vi "ADC_Abort.vi"(8 "error in (no error)":errorcluster) -> (0 "error out":errorcluster, 3 "function return":i16)   [LabVIEW 2013, in "MeasurmentRoutines.lvlib"]
doc: "Description: This routine aborts a running measurement. Any measured datais lost. It is not required to abort a running measurement before starting a new one, ADC_Start does this already.\nInput: -\nOutput: Return value E_NOT_INITIALIZED | E_NO_ERRORS | E_NO_HARDWARE\n\nFunction prototype: word ADC_Abort( void )\n\n\nshort int ADC_Abort ( void );"
uses:
  MeasurmentRoutines.lvlib
  hs3.dll
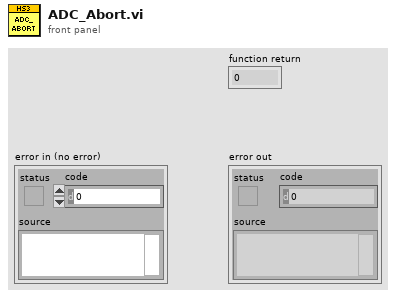
[diagram p1: front panel]
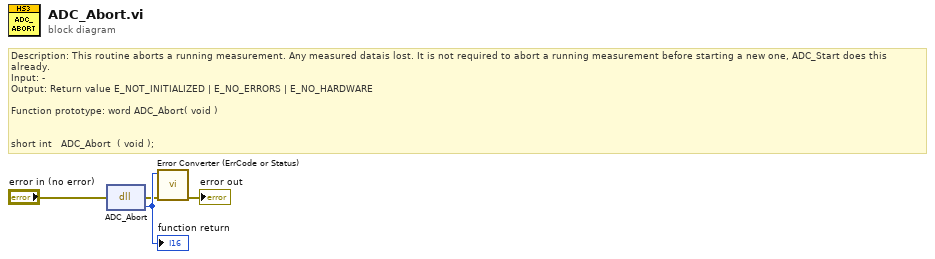
[diagram p0: block diagram]
diagram:
  # "Description: This routine aborts a running measurement. Any measured datais lost. It is not required to abort a running measurement before starting a new one, ADC_Start does this already.\nInput: -\nOutput: Return value E_NOT_INITIALIZED | E_NO_ERRORS | E_NO_HARDWARE\n\nFunction prototype: word ADC_Abort( void )\n\n\nshort int \t\tADC_Abort\t\t( void );"
  n1 = dll-call lib="C:/Documents and Settings/admin/Pulpit/HS3 LabViewLib/HS3_WRAPPER/hs3.*" fn="ADC_Abort"(error in="error in (no error)") -> (error out=w2:errorcluster, w4:i16)  [unwired: 2 in, 1 out]
  "function return" <- w4
  n2 = call "Error Converter (ErrCode or Status).vi"("error in (no error)"=w2, "error code"=w4) -> ("error out"=→"error out":errorcluster)  [unwired: 9 in]
